vi "Download from vi.vi"(8 "Indent Level":i32, 10 "Parent tag":string, 11 "Gen Refnum":refnum<vi>) -> (1 "Ctrl Tag":string[](array[string]), 2 "Ctrl Ref":refnum<vi>[](array[refnum]), 3 "appended array":T1(array[cluster]))   [LabVIEW 2021, in "Tree.lvlib" / "Tree.lvclass"]
uses:
  Tree.lvclass
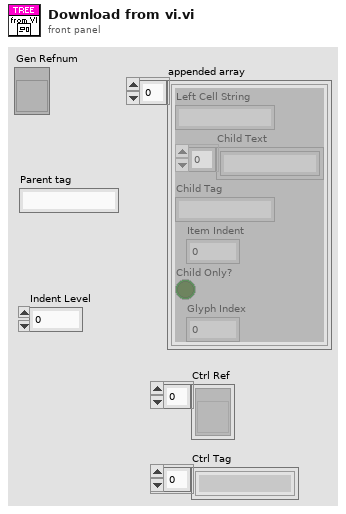
[diagram p1: front panel]
types:
  T1 = cluster{"Left Cell String":string, "Child Text":string[], "Child Tag":string, "Item Indent":i32, "Child Only?":bool, "Glyph Index":i32}[]
  T2 = cluster{"Left Cell String":string, "Child Text":string[], "Child Tag":string, "Item Indent":i32, "Child Only?":bool, "Glyph Index":i32}
  T3 = cluster{"Combo Box":string, "Strings [4]":string[]}
  T4 = cluster{"Combo Box":string, "Strings [4]":string[]}[]
  T5 = cluster{"Combo Box":string, "Strings []":string[]}
  T6 = cluster{"Combo Box":string, "Strings []":string[]}[]
  T7 = cluster{"Combo Box":string, "Item Names":string[]}
  T8 = cluster{"Combo Box":string, "Item Names":string[]}[]
  T9 = cluster{"Combo Box":string, "ColHdrString":string[]}
  T10 = cluster{"Combo Box":string, "RowHdrs[]":string[]}
  T11 = cluster{"Combo Box":string, "RowHdrs[]":string[]}[]
  T12 = cluster{"Combo Box":string, "Column Headers[]":string[]}
  T13 = cluster{"Combo Box":string, "Row Headers[]":string[]}
  T14 = cluster{"Combo Box":string, "Row Headers[]":string[]}[]
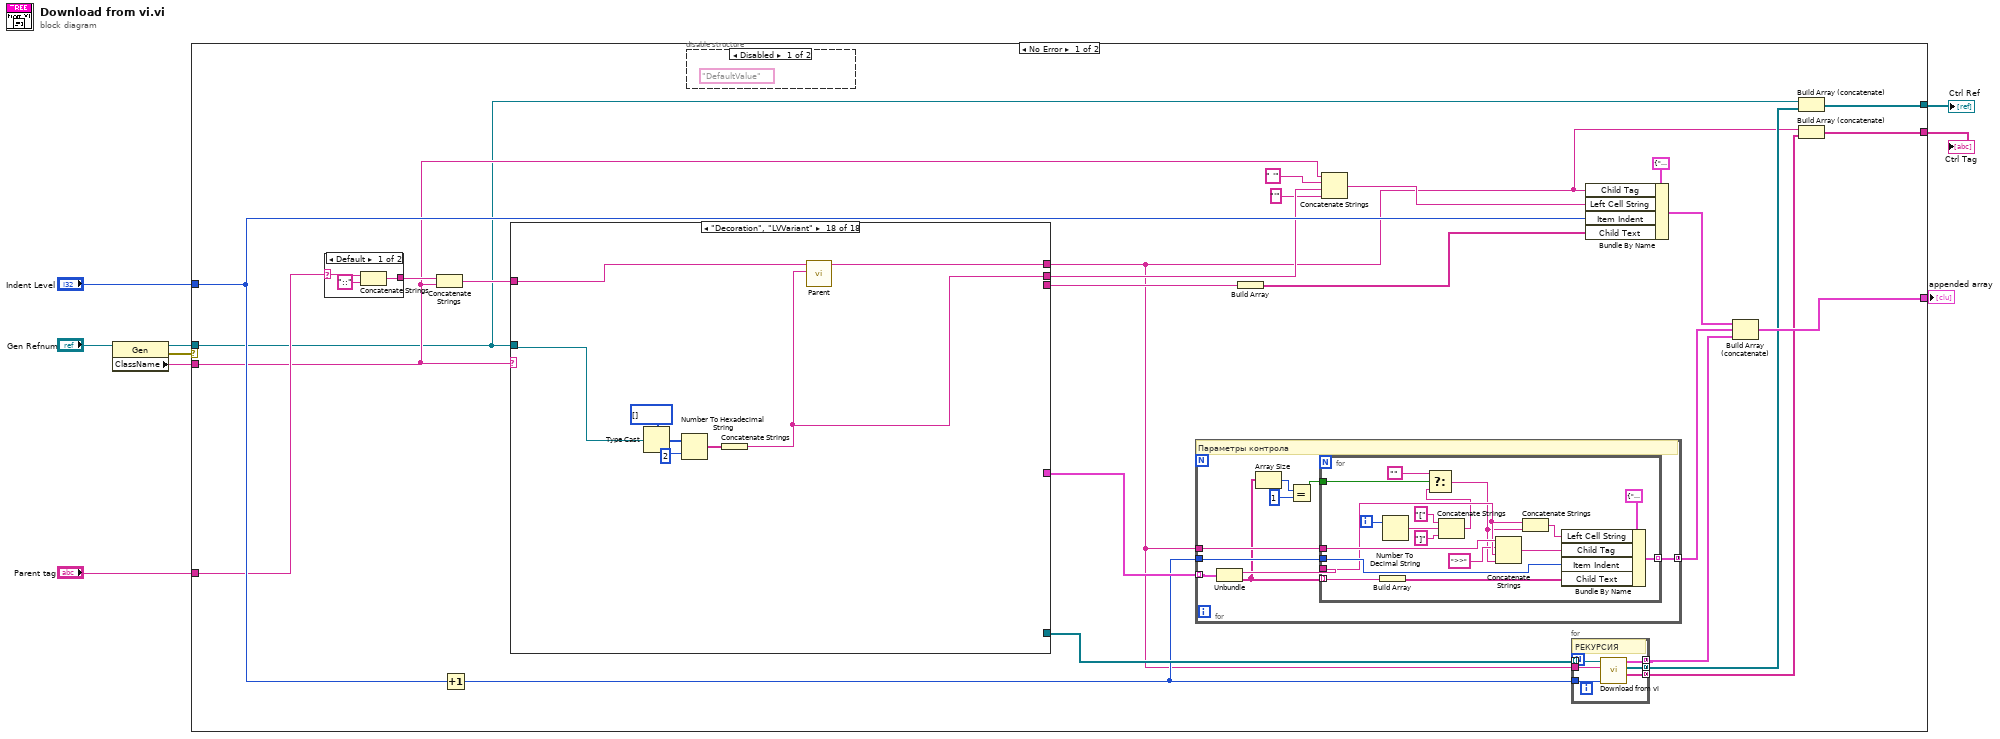
[diagram p0: block diagram]
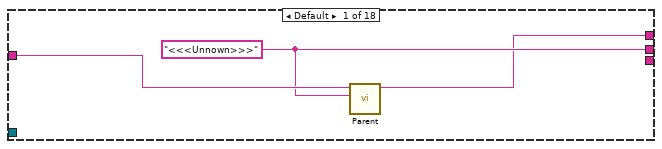
[diagram p4: hidden frame]
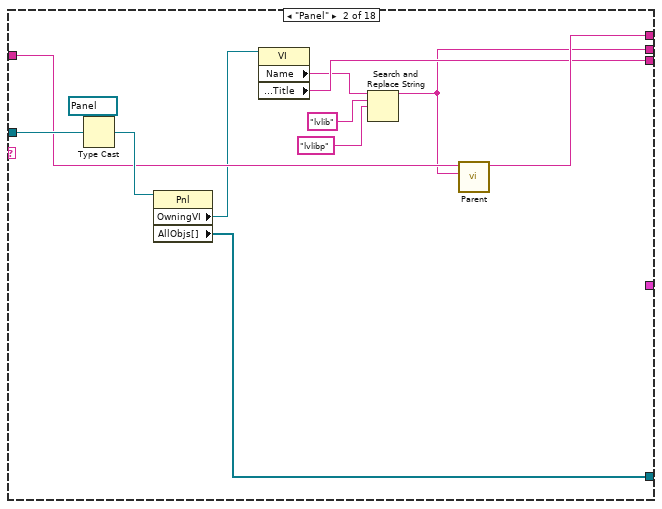
[diagram p5: hidden frame]
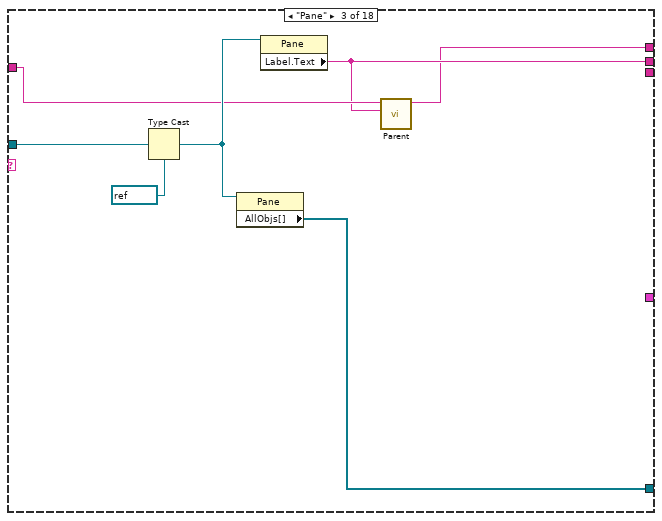
[diagram p6: hidden frame]
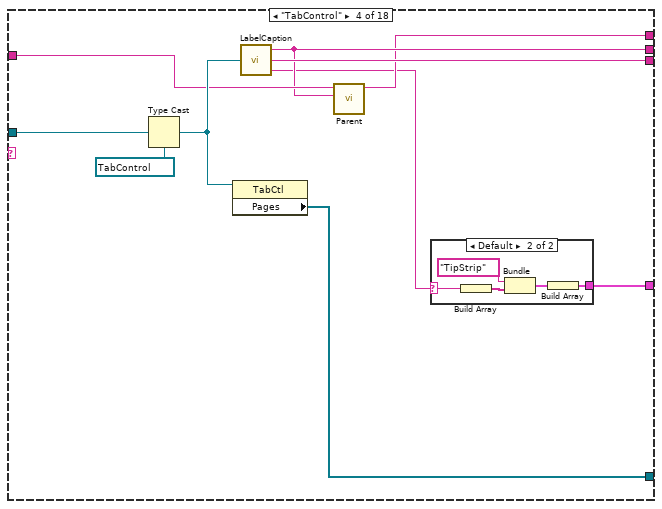
[diagram p7: hidden frame]
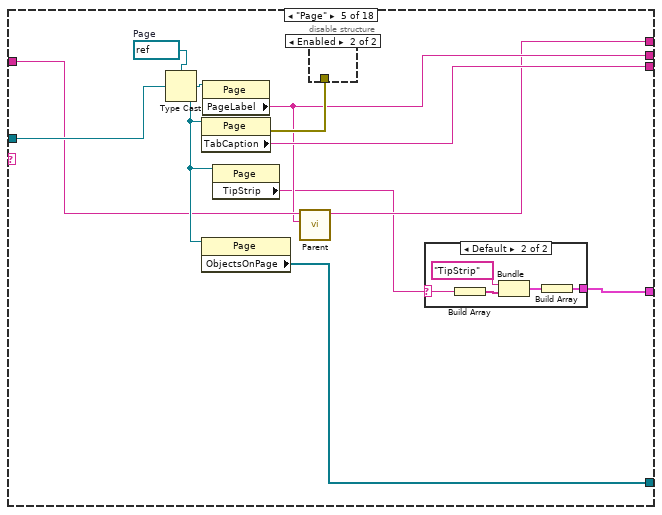
[diagram p9: hidden frame]
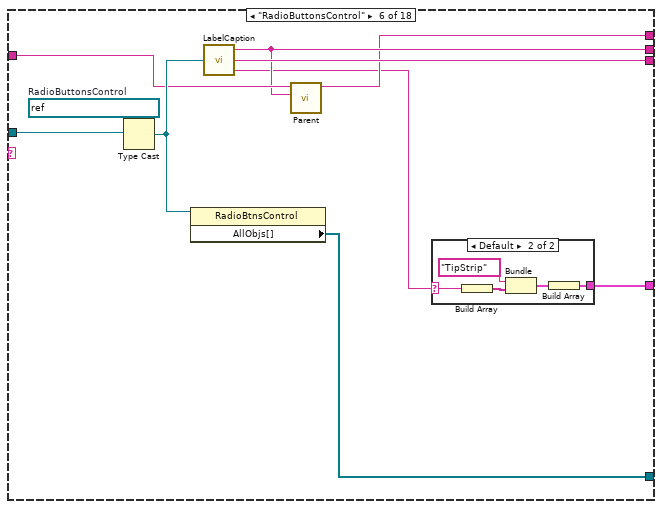
[diagram p12: hidden frame]
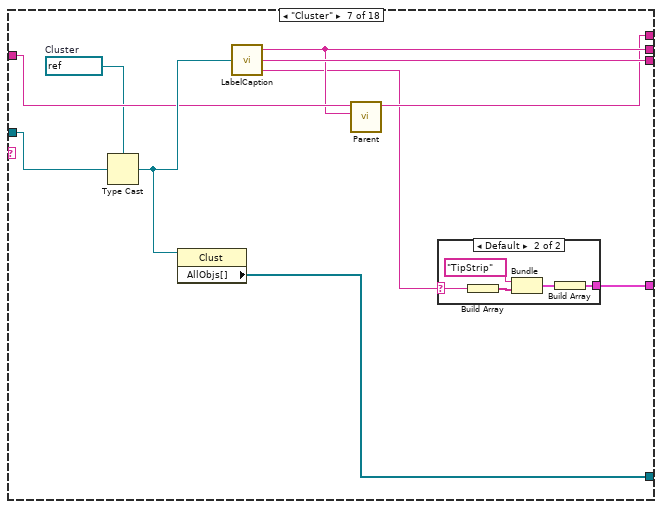
[diagram p14: hidden frame]
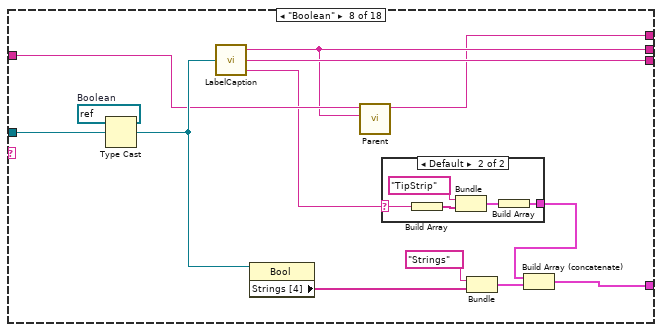
[diagram p16: hidden frame]
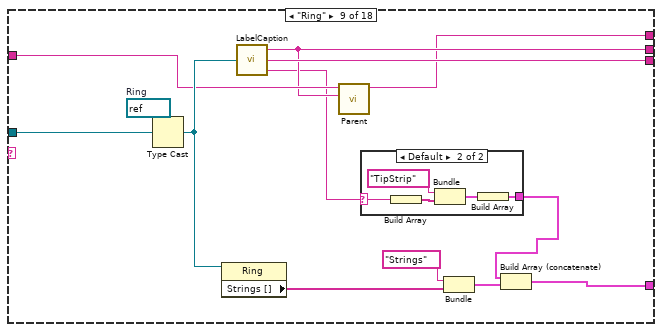
[diagram p18: hidden frame]
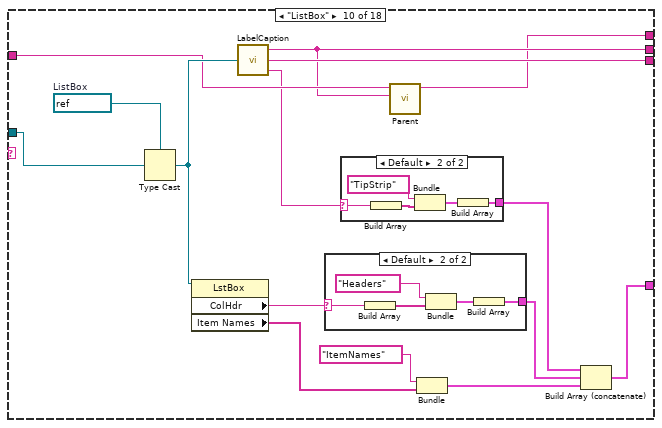
[diagram p20: hidden frame]
diagram:
  n1 = property class="Gen"(reference="Gen Refnum") -> (reference out=w8:refnum<vi>, error out=w5:errorcluster, "ClassName"=w4:string)  [unwired: 1 in]
  n2 = case shown="No Error" w5 {
    tunnel: w4 -> [w25 _]
    tunnel: w8 -> [w15 _]
    tunnel: [w34 _] -> w7
    tunnel: "Indent Level" -> [w29 _]
    tunnel: "Parent tag" -> [w28 _]
    tunnel: [w14 _] -> w2
    tunnel: [w12 _] -> w1
    frame No Error {
      n3 = case shown="Default" w28 {
        selector: w28 -> [w70 w71]
        tunnel: [w68 w71] -> w27
        frame Default {
          n4 = Concatenate Strings(w70, "::" ("string")) -> (w68:string)
        }
        frame "" {
        }
      }
      n5 = Concatenate Strings(w27, w25) -> (w26:string)
      n6 = Increment(x=w29) -> (x+1=w16:i32)
      n7 = case shown="\"Decoration\", \"LVVariant\"" w25 {
        tunnel: w15 -> [_ w86 w93 w103 w119 w134 w149 w167 w185 w205 w228 w246 w268 w289 w309 w326 w341 w344]
        tunnel: [w73 w75 w89 w99 w113 w130 w145 w163 w181 w200 w224 w243 w262 w283 w304 w322 w332 w343] -> w23
        tunnel: [_ w80 _ w101 w116 w132 w147 w165 w182 w203 w226 w245 w266 w287 w308 w324 w339 _] -> w31
        tunnel: w26 -> [w74 w83 w90 w100 w114 w131 w146 w164 w183 w201 w225 w244 w264 w285 w306 w323 w340 w350]
        tunnel: [w72 w82 w88 w98 w112 w129 w144 w157 w175 w193 w223 w242 w263 w284 w305 w320 w338 w349] -> w10
        tunnel: [_ _ _ w94 w109 w125 w140 w158 w176 w197 w221 w239 w255 w279 w297 w316 _ _] -> w20
        tunnel: [_ w79 w87 w96 w111 w127 w142 _ _ _ _ _ _ _ _ w318 _ _] -> w18
        frame Default {
          w73 = "<<<Unnown>>>" ("Label")
          n8 = call "Parent.vi"("Label.Text"=w73, "Parent in"=w74) -> ("Parent out"=w72:string)  [unwired: 9 in]
        }
        frame "Panel" {
          n9 = Type Cast(type=refnum<vi> refnum ("Front Panel"), x=w86) -> (*(type *) &x=w84:refnum<vi>)
          n10 = property class="Pnl"(reference=w84) -> ("OwningVI"=w81:refnum<vi>, "AllObjs[]"=w79:refnum<vi>[])  [unwired: 1 in, 2 out]
          n11 = property class="VI"(reference=w81) -> ("Name"=w76:string, "Front Panel.Title"=w80:string)  [unwired: 1 in, 2 out]
          n12 = Search and Replace String(input string=w76, search string="lvlib", replace string="lvlibp" ("search string")) -> (result string=w75:string)  [unwired: 5 in, 3 out]
          n13 = call "Parent.vi"("Label.Text"=w75, "Parent in"=w83) -> ("Parent out"=w82:string)  [unwired: 9 in]
        }
        frame "Pane" {
          n14 = Type Cast(type=refnum<vi> refnum ("Pane"), x=w93) -> (*(type *) &x=w92:refnum<vi>)
          n15 = property class="Pane"(reference=w92) -> ("AllObjs[]"=w87:refnum<vi>[])  [unwired: 1 in, 2 out]
          n16 = property class="Pane"(reference=w92) -> ("Label.Text"=w89:string)  [unwired: 1 in, 2 out]
          n17 = call "Parent.vi"("Label.Text"=w89, "Parent in"=w90) -> ("Parent out"=w88:string)  [unwired: 9 in]
        }
        frame "TabControl" {
          n18 = Type Cast(type=refnum<vi> refnum ("Pane"), x=w103) -> (*(type *) &x=w102:refnum<vi>)
          n19 = property class="TabCtl"(reference=w102) -> ("Pages"=w96:refnum<vi>[])  [unwired: 1 in, 2 out]
          n20 = call "LabelCaption.vi"("Control in"=w102) -> ("Label.Text"=w99:string, "Caption.Text"=w101:string, "Tip Strip"=w95:string)  [unwired: 1 in]
          n21 = call "Parent.vi"("Label.Text"=w99, "Parent in"=w100) -> ("Parent out"=w98:string)  [unwired: 9 in]
          n22 = case shown="Default" w95 {
            selector: w95 -> [_ w104]
            tunnel: [_ w105] -> w94
            frame "" {
            }
            frame Default {
              n23 = Build Array(w104) -> (w107:string[])
              n24 = Bundle("Combo Box"="TipStrip", w107) -> (w106:cluster{"Combo Box":string, string[]})  [unwired: 1 in]
              n25 = Build Array(w106) -> (w105:cluster{"Combo Box":string, string[]}[])
            }
          }
        }
        frame "Page" {
          w118 = refnum<vi> refnum  # Page
          n26 = Type Cast(type=w118, x=w119) -> (*(type *) &x=w115:refnum<vi>)
          n27 = property class="Page"(reference=w115) -> (error out=w117:errorcluster, "TabCaption"=w116:string)  [unwired: 1 in, 1 out]
          n28 = property class="Page"(reference=w115) -> ("ObjectsOnPage"=w111:refnum<vi>[])  [unwired: 1 in, 2 out]
          n29 = property class="Page"(reference=w115) -> ("PageLabel"=w113:string)  [unwired: 1 in, 2 out]
          n30 = property class="Page"(reference=w115) -> ("TipStrip"=w110:string)  [unwired: 1 in, 2 out]
          n31 = call "Parent.vi"("Label.Text"=w113, "Parent in"=w114) -> ("Parent out"=w112:string)  [unwired: 9 in]
          n32 = disable-structure shown="Enabled" {
            disable-tunnel: w117 -> [_ _]
            frame Disabled {
            }
            frame Enabled {
            }
          }
          n33 = case shown="Default" w110 {
            selector: w110 -> [_ w120]
            tunnel: [_ w121] -> w109
            frame "" {
            }
            frame Default {
              n34 = Build Array(w120) -> (w123:string[])
              n35 = Bundle("Combo Box"="TipStrip", w123) -> (w122:cluster{"Combo Box":string, string[]})  [unwired: 1 in]
              n36 = Build Array(w122) -> (w121:cluster{"Combo Box":string, string[]}[])
            }
          }
        }
        frame "RadioButtonsControl" {
          w128 = refnum<vi> refnum  # RadioButtonsControl
          n37 = Type Cast(type=w128, x=w134) -> (*(type *) &x=w133:refnum<vi>)
          n38 = property class="RadioBtnsControl"(reference=w133) -> ("AllObjs[]"=w127:refnum<vi>[])  [unwired: 1 in, 2 out]
          n39 = call "LabelCaption.vi"("Control in"=w133) -> ("Label.Text"=w130:string, "Caption.Text"=w132:string, "Tip Strip"=w126:string)  [unwired: 1 in]
          n40 = call "Parent.vi"("Label.Text"=w130, "Parent in"=w131) -> ("Parent out"=w129:string)  [unwired: 9 in]
          n41 = case shown="Default" w126 {
            selector: w126 -> [_ w135]
            tunnel: [_ w136] -> w125
            frame "" {
            }
            frame Default {
              n42 = Build Array(w135) -> (w138:string[])
              n43 = Bundle("Combo Box"="TipStrip", w138) -> (w137:cluster{"Combo Box":string, string[]})  [unwired: 1 in]
              n44 = Build Array(w137) -> (w136:cluster{"Combo Box":string, string[]}[])
            }
          }
        }
        frame "Cluster" {
          w143 = refnum<vi> refnum  # Cluster
          n45 = Type Cast(type=w143, x=w149) -> (*(type *) &x=w148:refnum<vi>)
          n46 = property class="Clust"(reference=w148) -> ("AllObjs[]"=w142:refnum<vi>[])  [unwired: 1 in, 2 out]
          n47 = call "LabelCaption.vi"("Control in"=w148) -> ("Label.Text"=w145:string, "Caption.Text"=w147:string, "Tip Strip"=w141:string)  [unwired: 1 in]
          n48 = call "Parent.vi"("Label.Text"=w145, "Parent in"=w146) -> ("Parent out"=w144:string)  [unwired: 9 in]
          n49 = case shown="Default" w141 {
            selector: w141 -> [_ w150]
            tunnel: [_ w151] -> w140
            frame "" {
            }
            frame Default {
              n50 = Build Array(w150) -> (w153:string[])
              n51 = Bundle("Combo Box"="TipStrip", w153) -> (w152:cluster{"Combo Box":string, string[]})  [unwired: 1 in]
              n52 = Build Array(w152) -> (w151:cluster{"Combo Box":string, string[]}[])
            }
          }
        }
        frame "Boolean" {
          w162 = refnum<vi> refnum  # Boolean
          n53 = Type Cast(type=w162, x=w167) -> (*(type *) &x=w166:refnum<vi>)
          n54 = call "LabelCaption.vi"("Control in"=w166) -> ("Label.Text"=w163:string, "Caption.Text"=w165:string, "Tip Strip"=w156:string)  [unwired: 1 in]
          n55 = property class="Bool"(reference=w166) -> ("Strings [4]"=w160:string[])  [unwired: 1 in, 2 out]
          n56 = call "Parent.vi"("Label.Text"=w163, "Parent in"=w164) -> ("Parent out"=w157:string)  [unwired: 9 in]
          n57 = case shown="Default" w156 {
            selector: w156 -> [_ w168]
            tunnel: [_ w169] -> w155
            frame "" {
            }
            frame Default {
              n58 = Build Array(w168) -> (w171:string[])
              n59 = Bundle("Combo Box"="TipStrip", w171) -> (w170:cluster{"Combo Box":string, string[]})  [unwired: 1 in]
              n60 = Build Array(w170) -> (w169:cluster{"Combo Box":string, string[]}[])
            }
          }
          n61 = Bundle("Combo Box"="Strings", "Strings [4]"=w160) -> (w159:T3)  [unwired: 1 in]
          n62 = Build Array (concatenate)(w155, w159) -> (w158:T4)
        }
        frame "Ring" {
          w180 = refnum<vi> refnum  # Ring
          n63 = Type Cast(type=w180, x=w185) -> (*(type *) &x=w184:refnum<vi>)
          n64 = property class="Ring"(reference=w184) -> ("Strings []"=w177:string[])  [unwired: 1 in, 2 out]
          n65 = call "LabelCaption.vi"("Control in"=w184) -> ("Label.Text"=w181:string, "Caption.Text"=w182:string, "Tip Strip"=w174:string)  [unwired: 1 in]
          n66 = call "Parent.vi"("Label.Text"=w181, "Parent in"=w183) -> ("Parent out"=w175:string)  [unwired: 9 in]
          n67 = case shown="Default" w174 {
            selector: w174 -> [_ w186]
            tunnel: [_ w187] -> w173
            frame "" {
            }
            frame Default {
              n68 = Build Array(w186) -> (w189:string[])
              n69 = Bundle("Combo Box"="TipStrip", w189) -> (w188:cluster{"Combo Box":string, string[]})  [unwired: 1 in]
              n70 = Build Array(w188) -> (w187:cluster{"Combo Box":string, string[]}[])
            }
          }
          n71 = Bundle("Combo Box"="Strings", "Strings []"=w177) -> (w178:T5)  [unwired: 1 in]
          n72 = Build Array (concatenate)(w173, w178) -> (w176:T6)
        }
        frame "ListBox" {
          w199 = refnum<vi> refnum  # ListBox
          n73 = Type Cast(type=w199, x=w205) -> (*(type *) &x=w204:refnum<vi>)
          n74 = property class="LstBox"(reference=w204) -> ("ColHdr"=w202:string, "Item Names"=w195:string[])  [unwired: 1 in, 2 out]
          n75 = call "LabelCaption.vi"("Control in"=w204) -> ("Label.Text"=w200:string, "Caption.Text"=w203:string, "Tip Strip"=w192:string)  [unwired: 1 in]
          n76 = case shown="Default" w202 {
            selector: w202 -> [_ w215]
            tunnel: [_ w211] -> w198
            frame "" {
            }
            frame Default {
              n77 = Build Array(w215) -> (w213:string[])
              n78 = Bundle("Combo Box"="Headers", w213) -> (w212:cluster{"Combo Box":string, string[]})  [unwired: 1 in]
              n79 = Build Array(w212) -> (w211:cluster{"Combo Box":string, string[]}[])
            }
          }
          n80 = case shown="Default" w192 {
            selector: w192 -> [_ w206]
            tunnel: [_ w207] -> w191
            frame "" {
            }
            frame Default {
              n81 = Build Array(w206) -> (w209:string[])
              n82 = Bundle("Combo Box"="TipStrip", w209) -> (w208:cluster{"Combo Box":string, string[]})  [unwired: 1 in]
              n83 = Build Array(w208) -> (w207:cluster{"Combo Box":string, string[]}[])
            }
          }
          n84 = call "Parent.vi"("Label.Text"=w200, "Parent in"=w201) -> ("Parent out"=w193:string)  [unwired: 9 in]
          n85 = Bundle("Combo Box"="ItemNames", "Item Names"=w195) -> (w194:T7)  [unwired: 1 in]
          n86 = Build Array (concatenate)(w191, w198, w194) -> (w197:T8)
        }
        frame "String" {
          n87 = Type Cast(type=refnum<vi> refnum ("Type"), x=w228) -> (*(type *) &x=w217:refnum<vi>)
          n88 = invoke class="Str" method="Reinit To Default"(reference=w217) -> (reference out=w216:refnum<vi>)  [unwired: 2 in, 2 out]
          n89 = property class="Str"(reference=w216) -> ("Value"=w218:string)  [unwired: 1 in, 2 out]
          n90 = call "LabelCaption.vi"("Control in"=w217) -> ("Label.Text"=w224:string, "Caption.Text"=w226:string, "Tip Strip"=w219:string)  [unwired: 1 in]
          n91 = case shown="Default" w218 {
            selector: w218 -> [_ w230]
            tunnel: [_ w229] -> w222
            frame "" {
            }
            frame Default {
              n92 = Build Array(w230) -> (w231:string[])
              n93 = Bundle("Combo Box"="DefaultValue", w231) -> (w232:cluster{"Combo Box":string, string[]})  [unwired: 1 in]
              n94 = Build Array(w232) -> (w229:cluster{"Combo Box":string, string[]}[])
            }
          }
          n95 = case shown="Default" w219 {
            selector: w219 -> [_ w234]
            tunnel: [_ w235] -> w220
            frame "" {
            }
            frame Default {
              n96 = Build Array(w234) -> (w237:string[])
              n97 = Bundle("Combo Box"="TipStrip", w237) -> (w236:cluster{"Combo Box":string, string[]})  [unwired: 1 in]
              n98 = Build Array(w236) -> (w235:cluster{"Combo Box":string, string[]}[])
            }
          }
          n99 = call "Parent.vi"("Label.Text"=w224, "Parent in"=w225) -> ("Parent out"=w223:string)  [unwired: 9 in]
          n100 = Build Array (concatenate)(w220, w222) -> (w221:cluster{"Combo Box":string, string[]}[])
        }
        frame "ComboBox", "Digital", "Enum", "Knob", "Slide", "WaveformChart" {
          n101 = Type Cast(type=refnum<vi> refnum ("Front Panel"), x=w246) -> (*(type *) &x=w247:refnum<vi>)
          n102 = call "LabelCaption.vi"("Control in"=w247) -> ("Label.Text"=w243:string, "Caption.Text"=w245:string, "Tip Strip"=w240:string)  [unwired: 1 in]
          n103 = case shown="Default" w240 {
            selector: w240 -> [_ w248]
            tunnel: [_ w249] -> w239
            frame "" {
            }
            frame Default {
              n104 = Build Array(w248) -> (w251:string[])
              n105 = Bundle("Combo Box"="TipStrip", w251) -> (w250:cluster{"Combo Box":string, string[]})  [unwired: 1 in]
              n106 = Build Array(w250) -> (w249:cluster{"Combo Box":string, string[]}[])
            }
          }
          n107 = call "Parent.vi"("Label.Text"=w243, "Parent in"=w244) -> ("Parent out"=w242:string)  [unwired: 9 in]
        }
        frame "TreeControl" {
          n108 = Type Cast(type=refnum<vi> refnum ("Front Panel"), x=w268) -> (*(type *) &x=w265:refnum<vi>)
          n109 = property class="Tree"(reference=w265) -> ("ColHdrString"=w257:string[], "RowHdrs[]"=w256:string[])  [unwired: 1 in, 2 out]
          n110 = call "LabelCaption.vi"("Control in"=w265) -> ("Label.Text"=w262:string, "Caption.Text"=w266:string, "Tip Strip"=w254:string)  [unwired: 1 in]
          n111 = call "Parent.vi"("Label.Text"=w262, "Parent in"=w264) -> ("Parent out"=w263:string)  [unwired: 9 in]
          n112 = Bundle("Combo Box"="Headers", "ColHdrString"=w257) -> (w260:T9)  [unwired: 1 in]
          n113 = Bundle("Combo Box"="Rows", "RowHdrs[]"=w256) -> (w258:T10)  [unwired: 1 in]
          n114 = case shown="Default" w254 {
            selector: w254 -> [_ w269]
            tunnel: [_ w270] -> w253
            frame "" {
            }
            frame Default {
              n115 = Build Array(w269) -> (w272:string[])
              n116 = Bundle("Combo Box"="TipStrip", w272) -> (w271:cluster{"Combo Box":string, string[]})  [unwired: 1 in]
              n117 = Build Array(w271) -> (w270:cluster{"Combo Box":string, string[]}[])
            }
          }
          n118 = Build Array (concatenate)(w253, w260, w258) -> (w255:T11)
        }
        frame "Table" {
          n119 = Type Cast(type=refnum<vi> refnum ("Front Panel"), x=w289) -> (*(type *) &x=w286:refnum<vi>)
          n120 = property class="Tbl"(reference=w286) -> ("Column Headers[]"=w281:string[], "Row Headers[]"=w277:string[])  [unwired: 1 in, 2 out]
          n121 = call "LabelCaption.vi"("Control in"=w286) -> ("Label.Text"=w283:string, "Caption.Text"=w287:string, "Tip Strip"=w275:string)  [unwired: 1 in]
          n122 = call "Parent.vi"("Label.Text"=w283, "Parent in"=w285) -> ("Parent out"=w284:string)  [unwired: 9 in]
          n123 = Bundle("Combo Box"="Headers", "Column Headers[]"=w281) -> (w280:T12)  [unwired: 1 in]
          n124 = Bundle("Combo Box"="Rows", "Row Headers[]"=w277) -> (w276:T13)  [unwired: 1 in]
          n125 = case shown="Default" w275 {
            selector: w275 -> [_ w290]
            tunnel: [_ w291] -> w274
            frame "" {
            }
            frame Default {
              n126 = Build Array(w290) -> (w293:string[])
              n127 = Bundle("Combo Box"="TipStrip", w293) -> (w292:cluster{"Combo Box":string, string[]})  [unwired: 1 in]
              n128 = Build Array(w292) -> (w291:cluster{"Combo Box":string, string[]}[])
            }
          }
          n129 = Build Array (concatenate)(w274, w280, w276) -> (w279:T14)
        }
        frame "MulticolumnListbox" {
          n130 = Type Cast(type=refnum<vi> refnum ("Front Panel"), x=w309) -> (*(type *) &x=w307:refnum<vi>)
          n131 = property class="MCListbox"(reference=w307) -> ("ColHdrString"=w303:string[], "RowHdrs[]"=w300:string[])  [unwired: 1 in, 2 out]
          n132 = call "LabelCaption.vi"("Control in"=w307) -> ("Label.Text"=w304:string, "Caption.Text"=w308:string, "Tip Strip"=w296:string)  [unwired: 1 in]
          n133 = call "Parent.vi"("Label.Text"=w304, "Parent in"=w306) -> ("Parent out"=w305:string)  [unwired: 9 in]
          n134 = Bundle("Combo Box"="Rows", "RowHdrs[]"=w300) -> (w298:T10)  [unwired: 1 in]
          n135 = Bundle("Combo Box"="Headers", "ColHdrString"=w303) -> (w299:T9)  [unwired: 1 in]
          n136 = case shown="Default" w296 {
            selector: w296 -> [_ w311]
            tunnel: [_ w312] -> w295
            frame "" {
            }
            frame Default {
              n137 = Build Array(w311) -> (w314:string[])
              n138 = Bundle("Combo Box"="TipStrip", w314) -> (w313:cluster{"Combo Box":string, string[]})  [unwired: 1 in]
              n139 = Build Array(w313) -> (w312:cluster{"Combo Box":string, string[]}[])
            }
          }
          n140 = Build Array (concatenate)(w295, w299, w298) -> (w297:T11)
        }
        frame "Array" {
          n141 = Type Cast(type=refnum<vi> refnum ("Front Panel"), x=w326) -> (*(type *) &x=w321:refnum<vi>)
          n142 = property class="Arr"(reference=w321) -> ("Array Element"=w319:refnum<vi>)  [unwired: 1 in, 2 out]
          n143 = call "LabelCaption.vi"("Control in"=w321) -> ("Label.Text"=w322:string, "Caption.Text"=w324:string, "Tip Strip"=w317:string)  [unwired: 1 in]
          n144 = Build Array(w319) -> (w318:refnum<vi>[])
          n145 = call "Parent.vi"("Label.Text"=w322, "Parent in"=w323) -> ("Parent out"=w320:string)  [unwired: 9 in]
          n146 = case shown="Default" w317 {
            selector: w317 -> [_ w327]
            tunnel: [_ w328] -> w316
            frame "" {
            }
            frame Default {
              n147 = Build Array(w327) -> (w330:string[])
              n148 = Bundle("Combo Box"="TipStrip", w330) -> (w329:cluster{"Combo Box":string, string[]})  [unwired: 1 in]
              n149 = Build Array(w329) -> (w328:cluster{"Combo Box":string, string[]}[])
            }
          }
        }
        frame "Text" {
          n150 = Type Cast(type=refnum<vi> refnum ("Front Panel"), x=w341) -> (*(type *) &x=w333:refnum<vi>)
          n151 = property class="Txt"(reference=w333) -> ("Text"=w339:string)  [unwired: 1 in, 2 out]
          n152 = Type Cast(type=u8[] [], x=w333) -> (*(type *) &x=w336:u8[])
          n153 = Number To Hexadecimal String(1:i16 2 ("width (-)"), 2:w336) -> (0:w334:string[])
          n154 = Concatenate Strings(w334) -> (w332:string)
          n155 = call "Parent.vi"("Label.Text"=w332, "Parent in"=w340) -> ("Parent out"=w338:string)  [unwired: 9 in]
        }
        frame "Decoration", "LVVariant" {
          n156 = Type Cast(type=u8[] [], x=w344) -> (*(type *) &x=w347:u8[])
          n157 = Number To Hexadecimal String(1:i16 2 ("width (-)"), 2:w347) -> (0:w345:string[])
          n158 = Concatenate Strings(w345) -> (w343:string)
          n159 = call "Parent.vi"("Label.Text"=w343, "Parent in"=w350) -> ("Parent out"=w349:string)  [unwired: 9 in]
        }
      }
      n160 = disable-structure shown="Disabled" {
        frame Disabled {
          (unwired) "DefaultValue" ("Combo Box")
        }
        frame Enabled {
        }
      }
      n161 = for {
        tunnel: w10 -> [w49]
        tunnel: w20 -> [w48] mode=indexing
        tunnel: w16 -> [w46]
        tunnel: [w45] -> w19 mode=concatenating
        # "Параметры контрола"
        n162 = Unbundle(w48) -> ("Combo Box"=w47:string, "RowHdrs[]"=w44:string[])
        n163 = Array Size(array=w44) -> (size(s)=w43:i32)
        n164 = Equal?(x=w43, y=1) -> (x = y?=w41:bool)
        n165 = for {
          tunnel: w44 -> [w64] mode=indexing
          tunnel: w46 -> [w66]
          tunnel: [w65] -> w45 mode=indexing
          tunnel: w47 -> [w55]
          tunnel: w49 -> [w56]
          tunnel: w41 -> [w53]
          i -> [w61]
          n166 = Build Array(w64) -> (w63:string[])
          n167 = Number To Decimal String(number=w61) -> (decimal integer string=w59:string)  [unwired: 1 in]
          n168 = Concatenate Strings("[" ("string"), w59, "]" ("string")) -> (w52:string)
          n169 = Select(t="", s=w53, f=w52) -> (s? t:f=w50:string)
          n170 = Concatenate Strings(w56, ">>" ("string"), w55, w50) -> (w58:string)
          n171 = Concatenate Strings(w55, w50) -> (w57:string)
          n172 = Bundle By Name(cluster=T2 {"Left Cell String"="", "Child Text"=[], "Child Tag"="", "Item Indent"=0, "Child Only?"=FALSE, "Glyph Index"=0} ("Item"), "Left Cell String"=w57, "Child Tag"=w58, "Item Indent"=w66, "Child Text"=w63) -> (w65:T2)
        }
      }
      n173 = Build Array(w31) -> (w30:string[])
      n174 = Concatenate Strings(w25, " '" ("string"), w23, "'" ("string")) -> (w21:string)
      n175 = for {
        tunnel: w18 -> [w40] mode=indexing
        tunnel: [w39] -> w17 mode=concatenating
        tunnel: w16 -> [w38]
        tunnel: w10 -> [w37]
        tunnel: [w36] -> w13 mode=concatenating
        tunnel: [w35] -> w11 mode=concatenating
        # "РЕКУРСИЯ"
        n176 = call "Download from vi.vi"("Indent Level"=w38, "Parent tag"=w37, "Gen Refnum"=w40) -> ("Ctrl Tag"=w35:string[], "Ctrl Ref"=w36:refnum<vi>[], "appended array"=w39:T1)  [unwired: 6 in]
      }
      n177 = Bundle By Name(cluster=T2 {"Left Cell String"="", "Child Text"=[], "Child Tag"="", "Item Indent"=0, "Child Only?"=FALSE, "Glyph Index"=0} ("Item"), "Child Tag"=w10, "Left Cell String"=w21, "Item Indent"=w29, "Child Text"=w30) -> (w32:T2)
      n178 = Build Array (concatenate)(w32, w19, w17) -> (w34:T1)
      n179 = Build Array (concatenate)(w15, w13) -> (w14:refnum<vi>[])
      n180 = Build Array (concatenate)(w10, w11) -> (w12:string[])
    }
    frame Error {
    }
  }
  "appended array" <- w7
  "Ctrl Ref" <- w2
  "Ctrl Tag" <- w1
